vi "ble_discover_handle_table_mod.vi"(6 "Connection Status":T1={"MAC Address"="", "cnx handle"=0, "cnx flags"=0, "Address Type"=125, "Connection Interval (ms)"=125, "Timeout(ms)"=125, "Latency"=0, "bonding handle"=0} {"Address Type" items=["Public", "Random"]}, 8 "error in (no error)":errorcluster, 11 "COM Bluegiga in":refnum<visa-resource-name>) -> (0 "error out":errorcluster, 1 "Handle description":string[](array[string]), 2 "Handle table":string[][](array[string]), 3 "COM Bluegiga out":refnum<visa-resource-name>)   [LabVIEW 2016]
doc: "This VI has been modified by Frax as a workaround for a bug in the original API. It provides as output the correct Handle table formatted as Handle - Service - Attribute of the service. It even provides a \"Handle description array\" that helps in the interpretation of the Handle Table"
uses:
  <vilib>/BLE/type_def/connection_status_bundle.ctl
  <vilib>/BLE/type_def/address_type.ctl
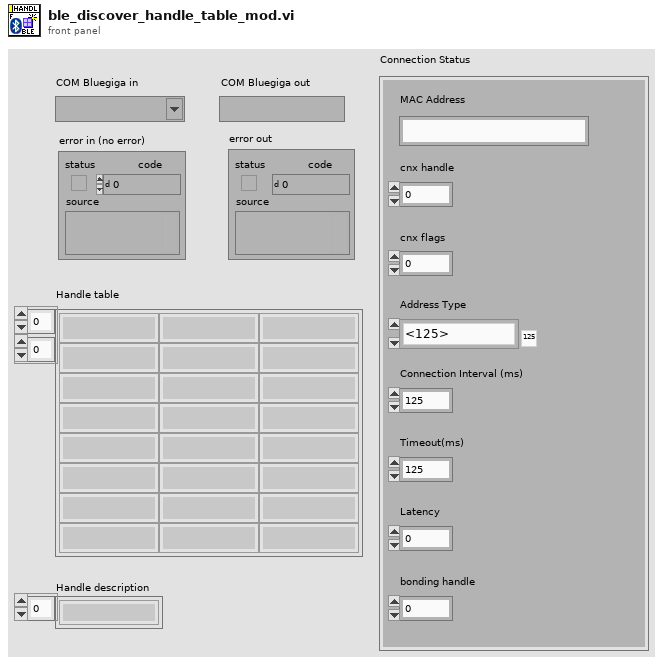
[diagram p1: front panel]
types:
  T1 = typedef "connection_status_bundle.ctl" = cluster{"MAC Address":string, "cnx handle":u8, "cnx flags":u8, "Address Type":T2, "Connection Interval (ms)":u16, "Timeout(ms)":u16, "Latency":u16, "bonding handle":u8}
  T2 = typedef "address_type.ctl" = u8
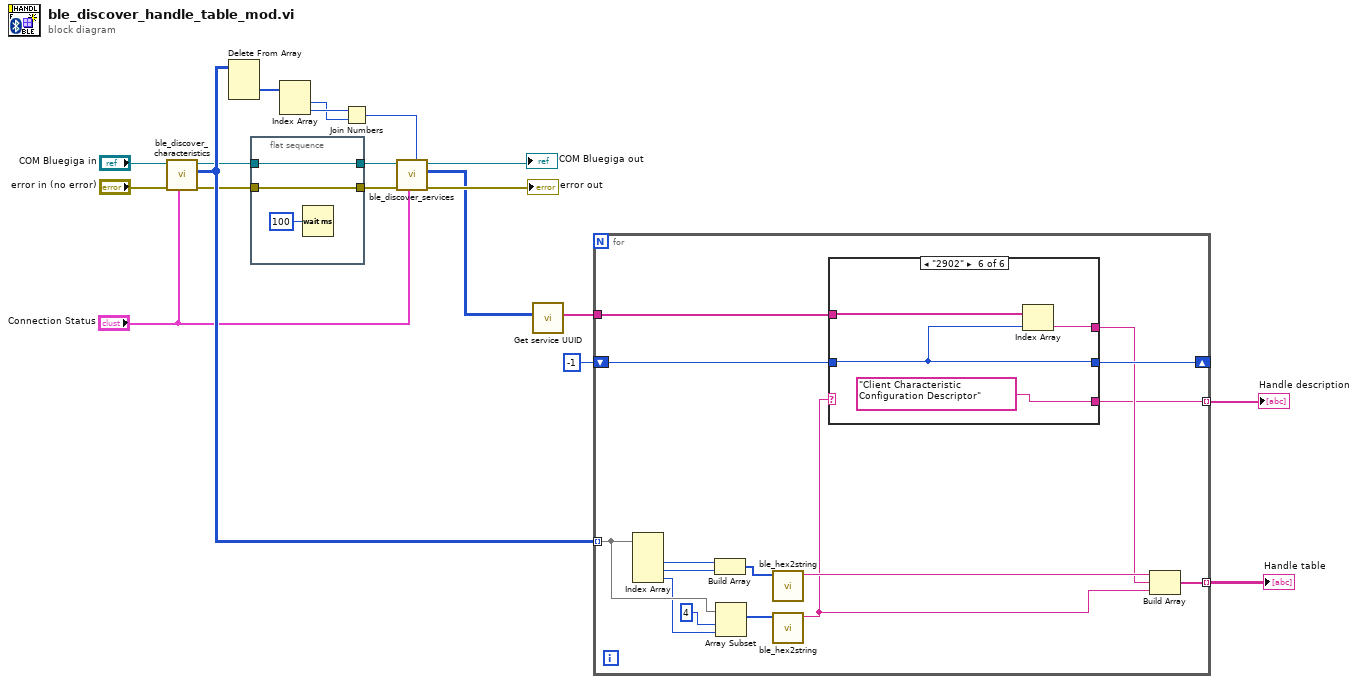
[diagram p0: block diagram]
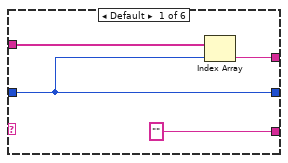
[diagram p2: hidden frame]
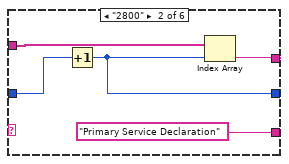
[diagram p3: hidden frame]
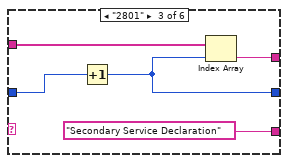
[diagram p4: hidden frame]
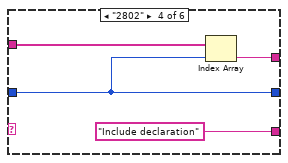
[diagram p5: hidden frame]
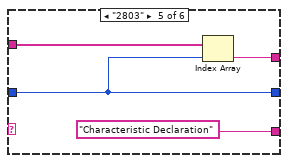
[diagram p6: hidden frame]
diagram:
  n1 = call <vilib>:"ble_discover_characteristics.vi"("Connection Status"="Connection Status", "error in (no error)"="error in (no error)", "COM Bluegiga in"="COM Bluegiga in") -> ("error out"=w1:errorcluster, "characteristics_info"=w11:u8[][], "COM Bluegiga out"=w3:refnum<visa-resource-name>)  [unwired: 6 in]
  n2 = Delete From Array(array=w11) -> (deleted portion=w15:u8[])  [unwired: 3 in, 1 out]
  n3 = flat-sequence {
    tunnel: [w21] -> w4
    tunnel: w3 -> [w21]
    tunnel: [w20] -> w2
    tunnel: w1 -> [w20]
    frame #0 {
      n4 = Wait (ms)(milliseconds to wait=u32 100) -> ()  [unwired: 1 out]
    }
  }
  n5 = Index Array(array=w15) -> (element #1=w13:u8, element #2=w14:u8)  [unwired: 2 in]
  n6 = Join Numbers(hi=w14, lo=w13) -> ((hi.lo)=w12:u16)
  n7 = call <vilib>:"ble_discover_services.vi"("Last Handle Number (0xFFFF)"=w12, "Connection Status"="Connection Status", "error in (no error)"=w2, "COM Bluegiga in"=w4) -> ("error out"=→"error out":errorcluster, "service_info"=w9:u8[][], "COM Bluegiga out"=→"COM Bluegiga out":refnum<visa-resource-name>)  [unwired: 5 in]
  n8 = call "Get service UUID.vi"("service_info"=w9) -> ("Service UUID list"=w8:string[])  [unwired: 9 in, 1 out]
  n9 = for {
    tunnel: w11 -> [w37] mode=indexing
    tunnel: [w35] -> w6 mode=indexing
    tunnel: w8 -> [w27]
    shift-right: [w25] -> _
    shift-left: -1 -> [w26]
    tunnel: [w23] -> w5 mode=indexing
    n10 = Index Array(array=w37) -> (element #2=w32:u8, element #3=w33:u8, element #4=w34:u8)  [unwired: 4 in, 1 out]
    n11 = Build Array(w32, w33) -> (w30:u8[])
    n12 = Array Subset(array=w37, index=4, length=w34) -> (w31:u8[])
    n13 = call <vilib>:"ble_hex2string.vi"("Byte Array IN (index0 LS byte)"=w30) -> ("HEX string OUT"=w29:string)  [unwired: 10 in]
    n14 = call <vilib>:"ble_hex2string.vi"("Byte Array IN (index0 LS byte)"=w31) -> ("HEX string OUT"=w28:string)  [unwired: 10 in]
    n15 = case shown="\"2902\"" w28 {
      tunnel: w27 -> [w41 w46 w51 w54 w58 w62]
      tunnel: w26 -> [w40 w45 w49 w53 w57 w61]
      tunnel: [w40 w42 w47 w53 w57 w61] -> w25
      tunnel: [w39 w44 w50 w52 w56 w60] -> w24
      tunnel: ["" "Primary Service Declaration" "Secondary Service Declaration" "Include declaration" "Characteristic Declaration" "Client Characteristic Configuration Descriptor"] -> w23
      frame Default {
        n16 = Index Array(array=w41, index=w40) -> (element=w39:string)
      }
      frame "2800" {
        n17 = Increment(x=w45) -> (x+1=w42:i32)
        n18 = Index Array(array=w46, index=w42) -> (element=w44:string)
      }
      frame "2801" {
        n19 = Increment(x=w49) -> (x+1=w47:i32)
        n20 = Index Array(array=w51, index=w47) -> (element=w50:string)
      }
      frame "2802" {
        n21 = Index Array(array=w54, index=w53) -> (element=w52:string)
      }
      frame "2803" {
        n22 = Index Array(array=w58, index=w57) -> (element=w56:string)
      }
      frame "2902" {
        n23 = Index Array(array=w62, index=w61) -> (element=w60:string)
      }
    }
    n24 = Build Array(w29, w24, w28) -> (w35:string[])
  }
  "Handle table" <- w6
  "Handle description" <- w5
